vi "PH_IEEE1394Camera.PC set Brightness.vi"(0 "i ref in":refnum<vi>, 1 "No Info? (False)":bool, 2 "Brightness":dbl, 3 "Tip Strip":string, 5 "error in (no error)":errorcluster, 7 "Brightness writable? (True)":bool=TRUE) -> (14 "i ref out":refnum<vi>, 19 "error out":errorcluster)   [LabVIEW 2014, in "PH_IEEE1394Camera.lvlib"]
doc: "This VI sets the incoming value to own attributes and the GUI element."
uses:
  PH_IEEE1394Camera.lvlib
  PH_Common/PH_Common.lvlib
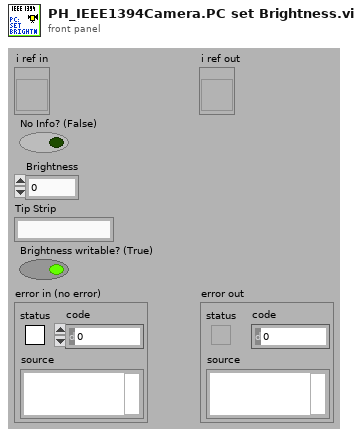
[diagram p1: front panel]
types:
  T1 = enum8{"Enabled", "Disabled", "Disabled and Grayed Out"}
  T2 = typedef "PH_IEEE1394Camera.lvlib/PH_IEEE1394Camera.i attribute.ctl" = cluster{"Gui Refs":cluster{"Brightness":refnum<vi>, "Shutter":refnum<vi>, "Gain":refnum<vi>, "Center of Gravity":refnum<vi>, "Supported Video Modes":refnum<vi>, "Trigger Polarity":refnum<vi>, "Trigger Mode":refnum<vi>, "Trigger Timeout":refnum<vi>, "Bit Depth":refnum<vi>, "Video Mode":refnum<vi>, "Top":refnum<vi>, "Bottom":refnum<vi>, "Left":refnum<vi>, "Right":refnum<vi>, "Set ROI to Maximum":refnum<vi>, "Camera Details":refnum<vi>, "Current Cam Attributes":refnum<vi>, "Attribute to set":refnum<vi>, "Num Value":refnum<vi>, "String Value":refnum<vi>, "Bool Value":refnum<vi>, "Set Cam Attribute":refnum<vi>}, "Cam":cluster{"IMAQ1394 Session":T3, "Camera Details":T4}, "Current Attributes":T5[], "Supported Video Modes ":cluster{"Video Mode":u32, "Video Mode Name":string}[], "Wanted Attributes":cluster{"Name":string, "Num Value":dbl, "String Value":string, "Boolean Value":bool}[], "Cam Attributes":T7}
  T3 = typedef "IMAQdx.ctl" = refnum<k21>
  T4 = typedef "PH_IEEE1394Camera.lvlib/PH_IEEE1394Camera.Cam Details.ctl" = cluster{"Model":string, "Serial Number":dbl, "Cam name (Machinery)":string, "Bus Type":string}
  T5 = typedef "PH_IEEE1394Camera.lvlib/PH_IEEE1394Camera.Cam Attribute.ctl" = cluster{"Information":cluster{"Type":T6, "Readable":bool, "Writable":bool, "Name":string}, "Num Value":dbl, "String Value":string, "Maximum":dbl, "Minimum":dbl, "Units":string, "Description":string, "EnumStrings[]":string[], "EnumValues[]":u32[], "Boolean Value":bool}
  T6 = typedef "NI_Vision_Acquisition_Software.lvlib/IMAQdx Attribute Type.ctl" = enum32{"U32", "I64", "DBL", "String", "Enum", "Bool", "Command"}
  T7 = typedef "PH_IEEE1394Camera.lvlib/PH_IEEE1394Camera.Relevant Cam Attributes.ctl" = cluster{"Video Mode":cluster{"Name":string, "Index":i32}, "Brightness":cluster{"Name":string, "Index":i32}, "Gain":cluster{"Name":string, "Index":i32}, "Shutter":cluster{"Name":string, "Index":i32}, "Trigger Pol":cluster{"Name":string, "Index":i32}, "Trigger Mode":cluster{"Name":string, "Index":i32}, "Timeout":cluster{"Name":string, "Index":i32}, "Bit Depth":cluster{"Name":string, "Index":i32}, "Pixel Bits":cluster{"Name":string, "Index":i32}, "Pixel Bytes":cluster{"Name":string, "Index":i32}, "Left":cluster{"Name":string, "Index":i32}, "Right":cluster{"Name":string, "Index":i32}, "Top":cluster{"Name":string, "Index":i32}, "Bottom":cluster{"Name":string, "Index":i32}}
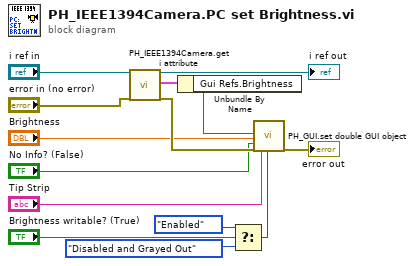
[diagram p0: block diagram]
diagram:
  n1 = call "PH_IEEE1394Camera.get i attribute.vi"("i ref in"="i ref in", "error in (no error)"="error in (no error)") -> ("i ref out"=→"i ref out":refnum<vi>, "i attribute"=w3:T2, "error out"=w10:errorcluster)  [unwired: 15 in]
  n2 = Unbundle By Name(w3) -> ("Gui Refs.Brightness"=w2:refnum<vi>)
  n3 = Select(t=T1."Enabled" ("Disabled"), s="Brightness writable? (True)", f=T1."Disabled and Grayed Out" ("Disabled")) -> (s? t:f=w5:T1)
  n4 = call "PH_GUI.set double GUI object.vi"("GUI object Ref"=w2, "value"="Brightness", "blinking (false)"="No Info? (False)", "error in (no error)"=w10, "Tip Strip [Empty]"="Tip Strip", "Disabled (Enabled)"=w5) -> ("error out"=→"error out":errorcluster)  [unwired: 13 in]
